vi "TazeASharg.vi"() -> ()   [LabVIEW 2022 SP3]
uses:
  StopControl.ctl
  StartControl.ctl
  ScoreIndicator.ctl
  TimeControl.ctl
  ComboIndicator.ctl
  NameControl.ctl
  FullHighscoreIndicator.ctl
  HighscoreIndicator.ctl
  FullHighScoreScoreIndicator.ctl
  HighscoreIndicatorYes.ctl
  ShargStates.ctl
  ShargTypeDef.ctl
  <vilib>/numeric/Random Number (Range) U64.vi
  <vilib>/numeric/sub_Random U32.vi
  <vilib>/MakerHub/LINX/Public/Utilities/Open Serial.vi
  <vilib>/MakerHub/LINX/Public/Sensors/Motion/Servo/Servo Open One Channel.vi
  <vilib>/MakerHub/LINX/Public/Sensors/Motion/Servo/Servo Close One Channel.vi
  <vilib>/MakerHub/LINX/LMH-LINX.lvlib
  <vilib>/MakerHub/LINX/Public/Sensors/Motion/Servo/Servo.lvlib
panel:
  out "High Score Scores":T1 caption="HIGH SCORE"
  out "High Score Names":T3 caption="HIGH SCORE"
  in  "Name":T5 caption="NAME"
  out "Overheat":bool
  out "COMBO":T6 format="%01d"
  out "TIME":T7 format="%02d"
  out "Hit?":bool
  out "SCORE":T8 format="%04d"
  in  "Start Game":T9
  in  "Stop Button":T10
  out "Energy":dbl(knob) caption="LASER ENERGY" scale=0.0..180.0
  # "HIGH SCORE"
  # "1."
  # "2."
  # "3."
  # "4."
  # "5."
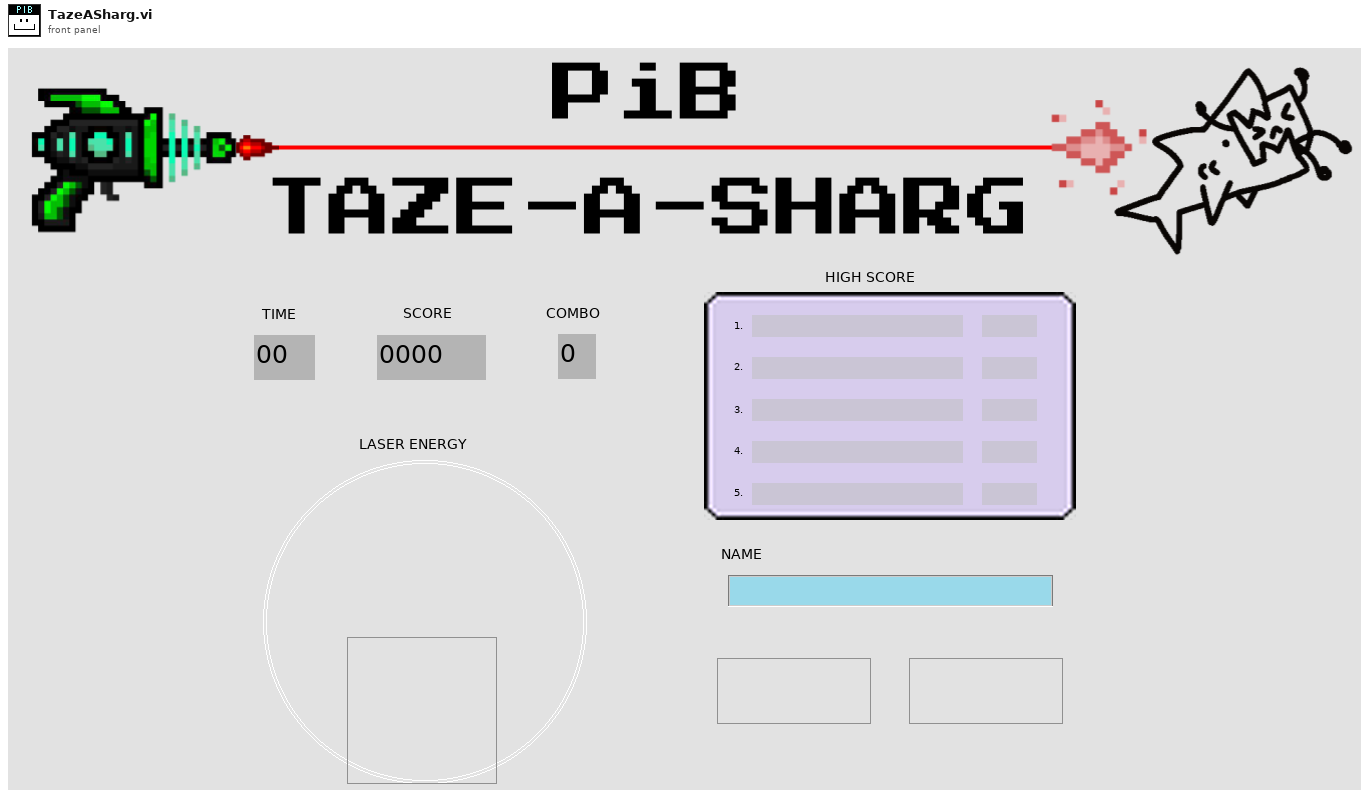
[diagram p1: front panel]
types:
  T1 = typedef "FullHighScoreScoreIndicator.ctl" = T2[]
  T2 = typedef "HighscoreIndicatorYes.ctl" = string
  T3 = typedef "FullHighscoreIndicator.ctl" = T4[]
  T4 = typedef "HighscoreIndicator.ctl" = string
  T5 = typedef "NameControl.ctl" = string
  T6 = typedef "ComboIndicator.ctl" = u32
  T7 = typedef "TimeControl.ctl" = u32
  T8 = typedef "ScoreIndicator.ctl" = u32
  T9 = typedef "StartControl.ctl" = bool
  T10 = typedef "StopControl.ctl" = bool
  T11 = cluster{"Target Up":bool, "Target Start Time":u32, "Target Up Time":u64, "Current Target":u64}
  T12 = cluster{"Laser Pin":u8, "Trigger Pin":u8, "Servo Pin":u8, "Photoresistor Pins":u8[], "RGB LED Pins":u8[]}
  T13 = typedef "ShargStates.ctl" = enum16{"Initialization", "Leaderboard", "Start Game", "Gameplay", "Update Final Score"}
  T14 = typedef "LMH-LINX.lvlib/LINX Ref.ctl" = cluster{"IO":T15, "Interface":T16, "LINX Device Config":T17}
  T15 = typedef "LMH-LINX.lvlib/Platform.ctl" = enum16{"Remote", "Local"}
  T16 = typedef "LMH-LINX.lvlib/Interface.ctl" = enum16{"Serial", "TCP"}
  T17 = typedef "LMH-LINX.lvlib/Device.lvlib/LINX Device Config.ctl" = cluster{"Interface":T16, "COM Port":refnum<visa-resource-name>, "TCP Configuration":T18, "Device Family":u8, "Device ID":u8, "Device Name":string, "TCP Ref":refnum<k5>, "Channels":T19}
  T18 = typedef "LMH-LINX.lvlib/Device.lvlib/TCP Config.ctl" = cluster{"IP Address":string, "Port":u16}
  T19 = typedef "LMH-LINX.lvlib/Channels.ctl" = cluster{"DI":u8[], "DO":u8[], "AI":u8[], "AO":u8[], "PWM":u8[], "QE":u8[], "UART":u8[], "I2C 2":u8[], "SPI":u8[], "CAN":u8[], "Servo":u8[], "AI Ref (V)":dbl, "AI Resolution (Bits)":u8, "AO Ref (V)":dbl, "AO Resolution (Bits)":u8}
  T20 = cluster{"Target Up":bool, "millisecond timer value":u32, "number":u64, "Current Target":u64}
  T21 = enum16{"open", "open or create", "create or replace", "create", "open (read-only)"}
  T22 = typedef "ShargTypeDef.ctl" = cluster{"Start Time":u32, "Score":u32, "Combo":u32, "RisingEdge":u32, "FallingEdge":u32, "Duration":u32, "Signal":i16, "NewTarget?":bool, "Username":string, "LastChannel":i32}
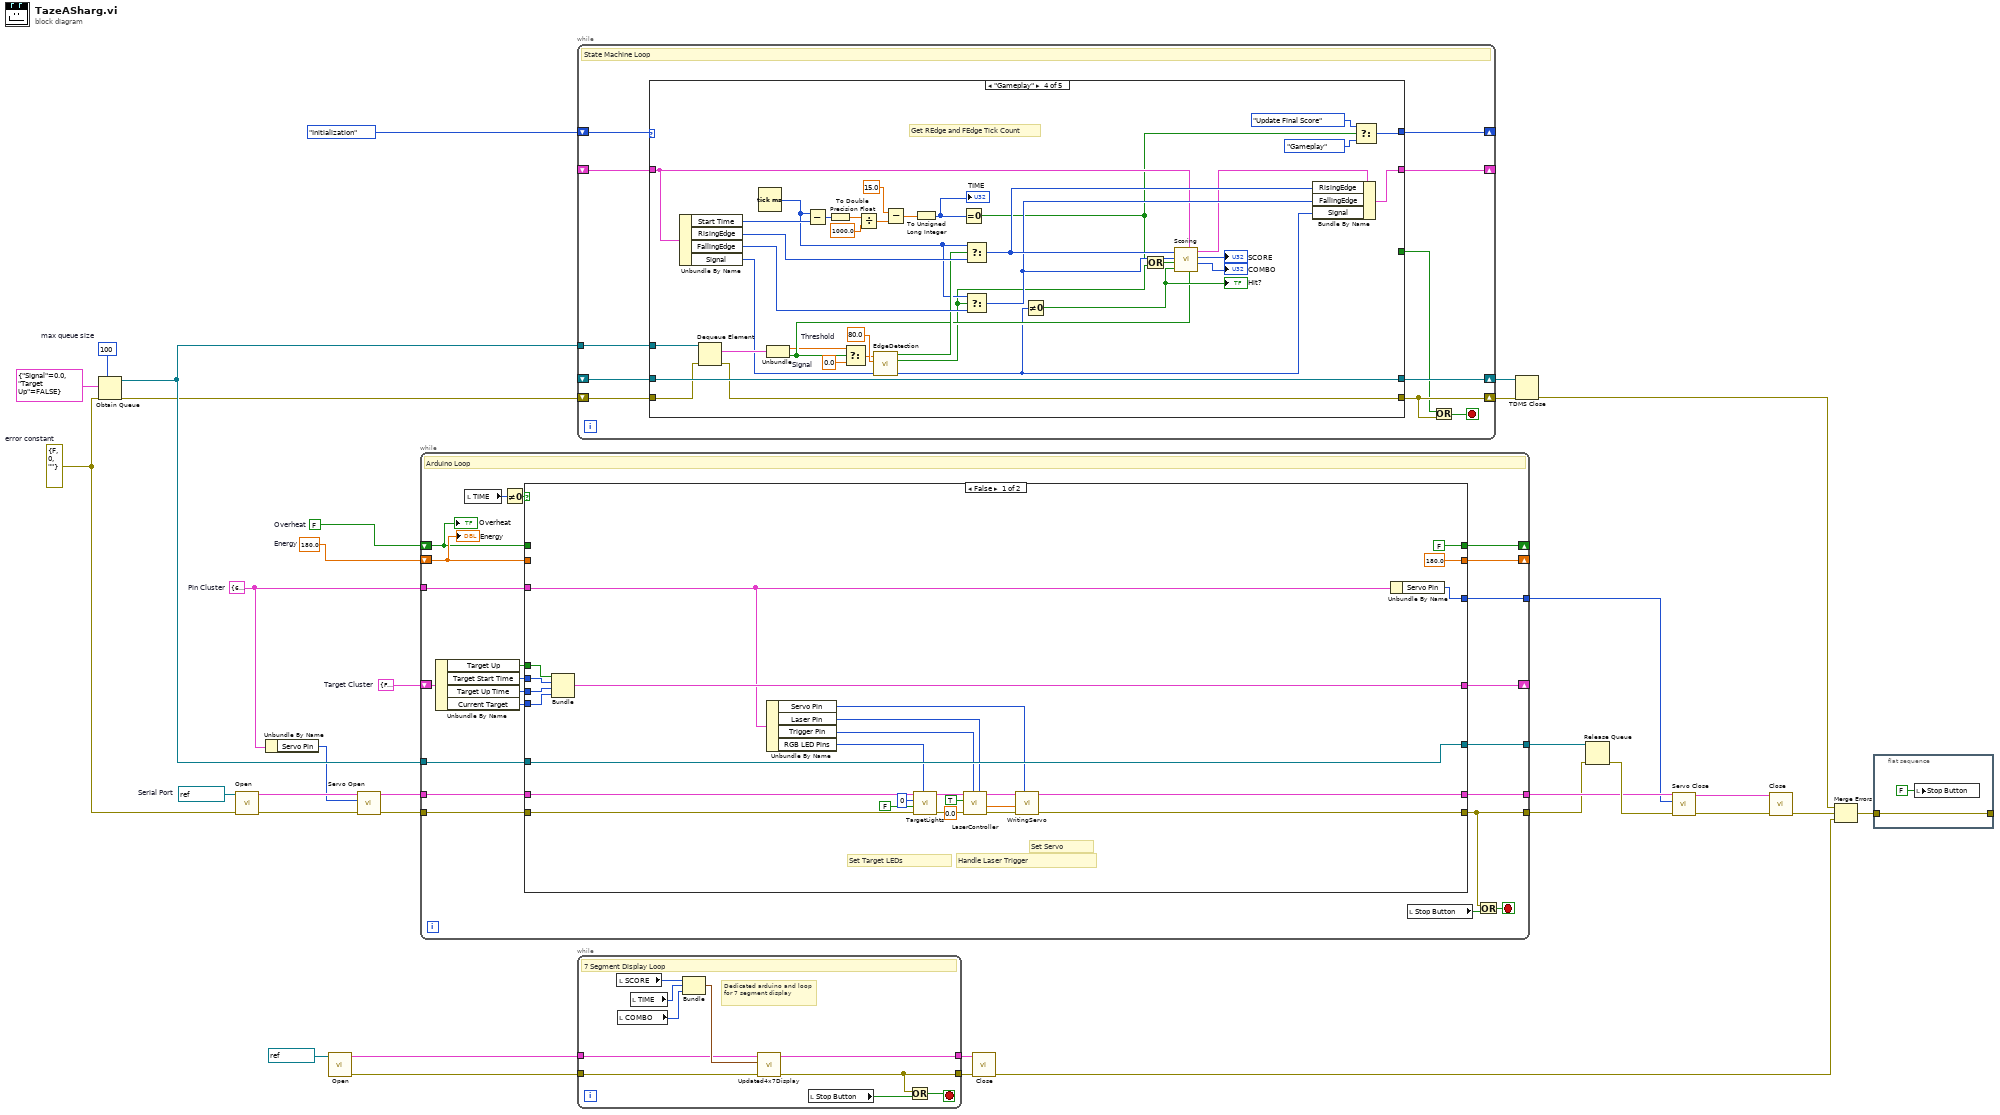
[diagram p0: block diagram]
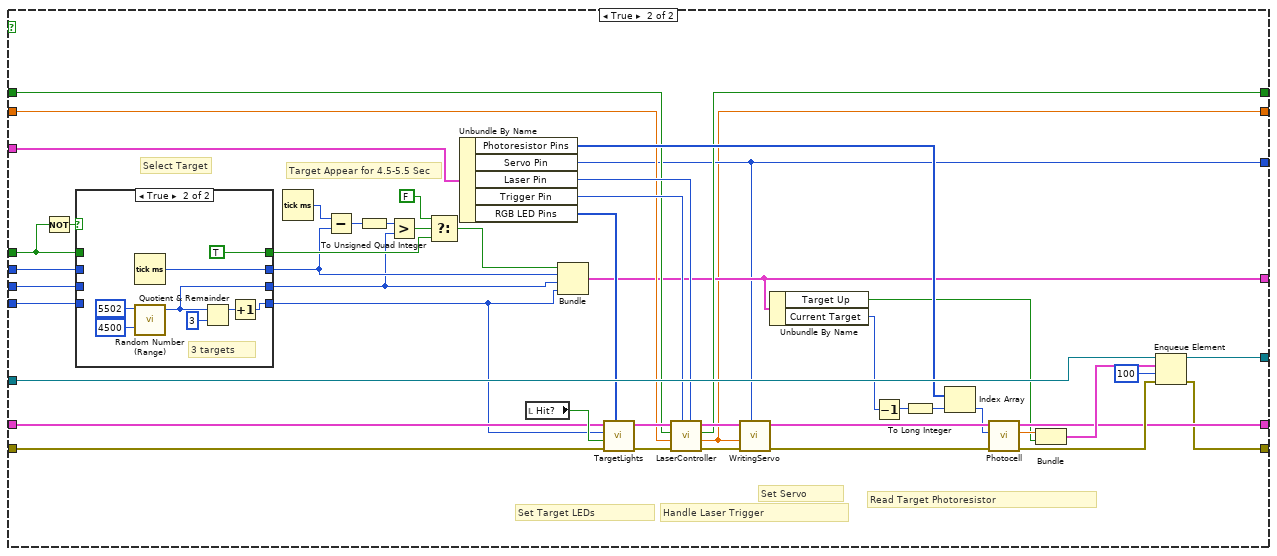
[diagram p2: hidden frame]
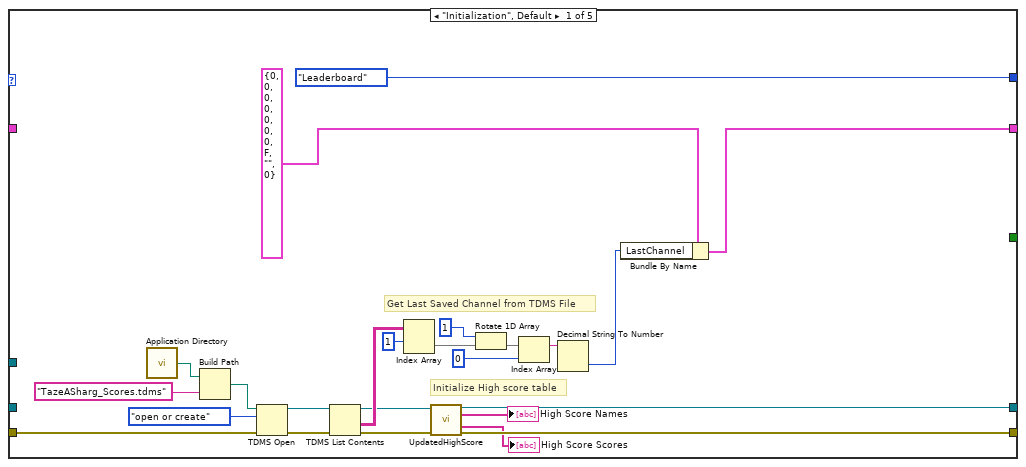
[diagram p4: hidden frame]
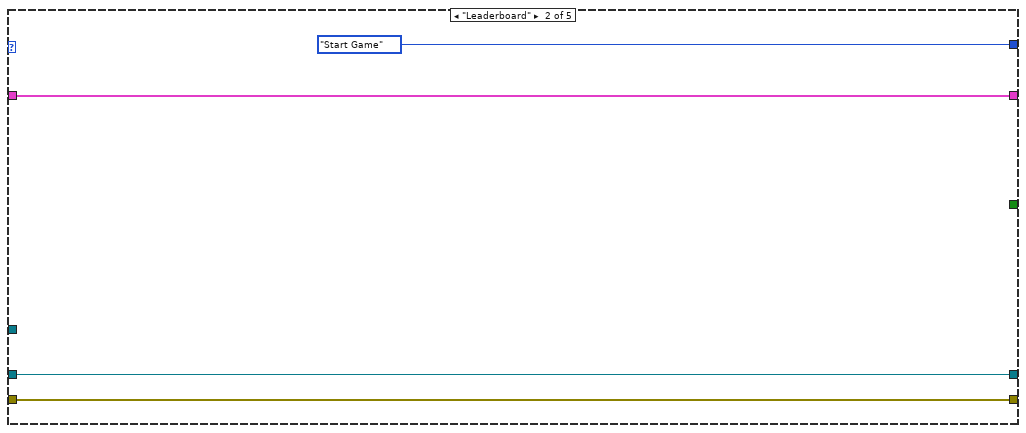
[diagram p5: hidden frame]
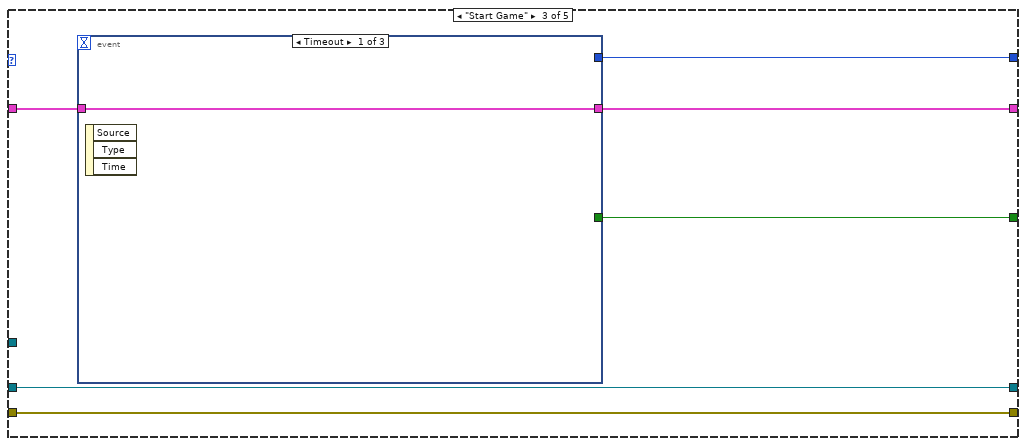
[diagram p6: hidden frame]
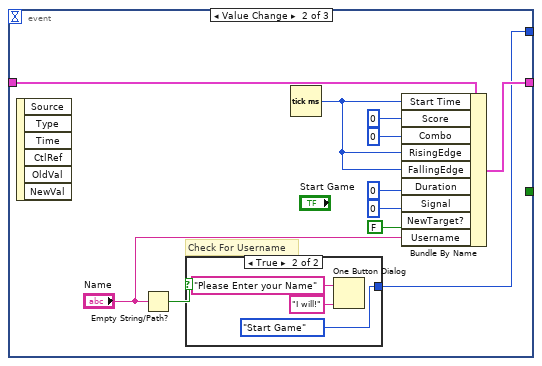
[diagram p7: hidden frame]
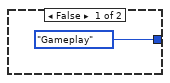
[diagram p8: hidden frame]
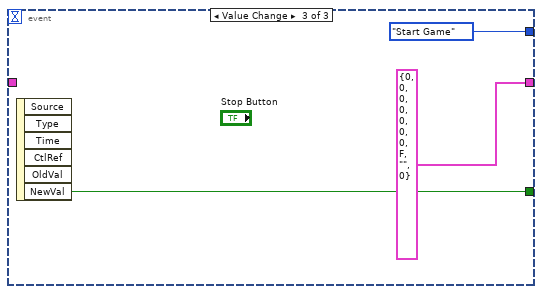
[diagram p9: hidden frame]
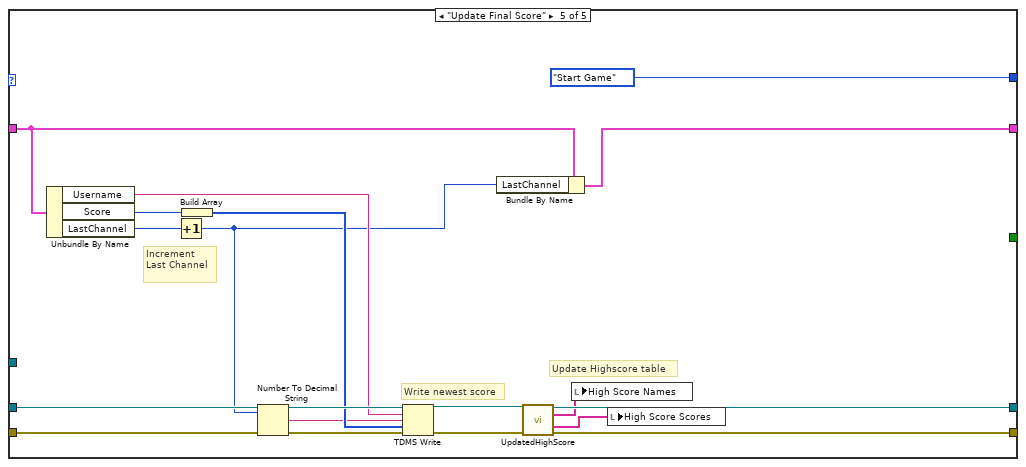
[diagram p10: hidden frame]
diagram:
  w5 = T11 {"Target Up"=FALSE, "Target Start Time"=0, "Target Up Time"=0, "Current Target"=0}  # Target Cluster
  w8 = 180.0  # Energy
  w9 = FALSE  # Overheat
  w2 = T12 {"Laser Pin"=6, "Trigger Pin"=3, "Servo Pin"=5, "Photoresistor Pins"=[0, 1, 2], "RGB LED Pins"=[22, 23, 24, 25, 26, 27]}  # Pin Cluster
  w30 = refnum<visa-resource-name> "COM8"  # Serial Port
  w31 = 100  # max queue size
  w10 = errorcluster {"status"=FALSE, "code"=0, "source"=""}  # error constant
  n1 = Obtain Queue(max queue size (-1, unlimited)=w31, element data type=cluster{"Signal":dbl, "Target Up":bool} {"Signal"=0.0, "Target Up"=FALSE}, error in (no error)=w10) -> (queue out=w33:refnum<queue>, error out=w11:errorcluster)  [unwired: 2 in, 1 out]
  n2 = call-poly <vilib>:"Open.vi"("Error In"=w10, "Serial Port"=w30) -> ("Error Out"=w27:errorcluster, "LINX Resource"=w29:T14)  [unwired: 7 in, 1 out]
  n3 = Unbundle By Name(w2) -> ("Servo Pin"=w1:u8)
  n4 = call-poly <vilib>:"Open.vi"("Serial Port"=refnum<visa-resource-name> "COM5") -> ("Error Out"=w20:errorcluster, "LINX Resource"=w21:T14)  [unwired: 8 in, 1 out]
  n5 = call-poly <vilib>:"Servo Open.vi"("Error In"=w27, "Servo Channel"=w1, "LINX Resource"=w29) -> ("Error Out"=w26:errorcluster, "LINX Resource"=w28:T14)  [unwired: 7 in]
  n6 = while {
    tunnel: w26 -> [w51]
    tunnel: w28 -> [w52]
    shift-right: [w48] -> _
    shift-left: w9 -> [w45]
    shift-right: [w47] -> _
    shift-left: w8 -> [w46]
    tunnel: w33 -> [w50]
    tunnel: w2 -> [w49]
    tunnel: [w44] -> w7
    tunnel: [w35] -> w3
    tunnel: [w43] -> w6
    shift-right: [w37] -> _
    shift-left: w5 -> [w42]
    tunnel: [w36] -> w4
    stop <- w54 stop-if-true
    # "Arduino Loop"
    n7 = Unbundle By Name(w42) -> ("Target Up"=w41:bool, "Target Start Time"=w40:u32, "Target Up Time"=w39:u64, "Current Target"=w38:u64)
    n8 = local read "TIME"() -> (w56:T7)
    n9 = Not Equal To 0?(x=w56) -> (x != 0?=w55:bool)
    n10 = case shown="False" w55 {
      tunnel: w40 -> [w79 w126]
      tunnel: w41 -> [w80 w125]
      tunnel: w38 -> [w77 w124]
      tunnel: w39 -> [w78 w123]
      tunnel: w52 -> [w66 w107]
      tunnel: w51 -> [w65 w106]
      tunnel: [w68 w105] -> w44
      tunnel: [w67 w104] -> w35
      tunnel: w50 -> [w81 w103]
      tunnel: w49 -> [w64 w101]
      tunnel: w46 -> [_ w96]
      tunnel: w45 -> [_ w95]
      tunnel: [FALSE ("Overheat Out") w94] -> w48
      tunnel: [180.0 ("Energy Out") w84] -> w47
      tunnel: [w81 w93] -> w43
      tunnel: [w76 w88] -> w37
      tunnel: [w75 w86] -> w36
      frame False {
        # "Set Servo"
        # "Handle Laser Trigger"
        # "Set Target LEDs"
        n11 = Bundle("Target Up"=w80, "Target Start Time"=w79, "Target Up Time"=w78, "Current Target"=w77) -> (w76:T11)  [unwired: 1 in]
        n12 = Unbundle By Name(w64) -> ("Servo Pin"=w60:u8, "Laser Pin"=w61:u8, "Trigger Pin"=w62:u8, "RGB LED Pins"=w63:u8[])
        n13 = call "TargetLights.vi"("DO Channels"=w63, "Error In"=w65, "Hit?"=FALSE, "Target Number"=u64 0, "LINX Resource"=w66) -> ("Error Out"=w71:errorcluster, "LINX Resource 2"=w72:T14)  [unwired: 5 in]
        n14 = call "LaserController.vi"("Laser Pin"=w61, "Trigger Pin"=w62, "Error In"=w71, "Energy In"=0.0, "Overheat In"=TRUE, "LINX Resource In"=w72) -> ("Error Out"=w74:errorcluster, "Energy Out"=w69:dbl, "LINX Resource Out"=w73:T14)  [unwired: 2 in, 1 out]
        n15 = call "WritingServo.vi"("Servo Pin"=w60, "error in (no error)"=w74, "Position"=w69, "LINX Resource in"=w73) -> ("error out"=w67:errorcluster, "LINX Resource out"=w68:T14)  [unwired: 6 in]
        n16 = Unbundle By Name(w64) -> ("Servo Pin"=w75:u8)
      }
      frame True {
        # "Set Servo"
        # "Read Target Photoresistor"
        # "Handle Laser Trigger"
        # "Set Target LEDs"
        # "Target Appear for 4.5-5.5 Sec"
        # "Select Target"
        n17 = Not(x=w125) -> (.not. x?=w122:bool)
        n18 = case shown="True" w122 {
          tunnel: [w134 TRUE] -> w128
          tunnel: [w135 w142] -> w91
          tunnel: [w133 w137] -> w89
          tunnel: w126 -> [w135 _]
          tunnel: w125 -> [w134 _]
          tunnel: w124 -> [w133 _]
          tunnel: [w132 w136] -> w90
          tunnel: w123 -> [w132 _]
          frame False {
          }
          frame True {
            # "3 targets"
            n19 = Tick Count (ms)() -> (millisecond timer value=w142:u32)
            n20 = call-poly <vilib>:"Random Number (Range).vi"("lower bound (0)"=u64 4500, "upper bound (100)"=u64 5502) -> ("number"=w136:u64)  [unwired: 9 in]
            n21 = Quotient & Remainder(x=w136, y=u64 3) -> (x-y*floor(x/y)=w139:u64)  [unwired: 1 out]
            n22 = Increment(x=w139) -> (x+1=w137:u64)
          }
        }
        n23 = Tick Count (ms)() -> (millisecond timer value=w131:u32)
        n24 = Subtract(x=w131, y=w91) -> (x-y=w130:u32)
        n25 = To Unsigned Quad Integer(1:w130) -> (0:w121:u64)
        n26 = Greater?(x=w121, y=w90) -> (0:w129:bool)
        n27 = Select(t=FALSE, s=w129, f=w128) -> (s? t:f=w92:bool)
        n28 = Unbundle By Name(w101) -> ("Photoresistor Pins"=w97:u8[], "Servo Pin"=w86:u8, "Laser Pin"=w98:u8, "Trigger Pin"=w99:u8, "RGB LED Pins"=w100:u8[])
        n29 = local read "Hit?"() -> (w114:bool)
        n30 = Bundle("Target Up"=w92, "millisecond timer value"=w91, "number"=w90, "Current Target"=w89) -> (w88:T20)  [unwired: 1 in]
        n31 = call "TargetLights.vi"("DO Channels"=w100, "Error In"=w106, "Hit?"=w114, "Target Number"=w89, "LINX Resource"=w107) -> ("Error Out"=w111:errorcluster, "LINX Resource 2"=w112:T14)  [unwired: 5 in]
        n32 = call "LaserController.vi"("Laser Pin"=w98, "Trigger Pin"=w99, "Error In"=w111, "Energy In"=w96, "Overheat In"=w95, "LINX Resource In"=w112) -> ("Error Out"=w120:errorcluster, "Energy Out"=w84:dbl, "Overheat Out"=w94:bool, "LINX Resource Out"=w119:T14)  [unwired: 2 in]
        n33 = call "WritingServo.vi"("Servo Pin"=w86, "error in (no error)"=w120, "Position"=w84, "LINX Resource in"=w119) -> ("error out"=w117:errorcluster, "LINX Resource out"=w116:T14)  [unwired: 6 in]
        n34 = Unbundle By Name(w88) -> ("Target Up"=w85:bool, "Current Target"=w87:u64)
        n35 = Decrement(x=w87) -> (x-1=w115:u64)
        n36 = To Long Integer(number=w115) -> (32bit integer=w113:i32)
        n37 = Index Array(array=w97, index=w113) -> (element=w102:u8)
        n38 = call <vilib>:"Photocell.vi"("Error In"=w117, "AI Channel"=w102, "LINX Resource"=w116) -> ("Error Out"=w118:errorcluster, "Value (0-100)"=w109:dbl, "LINX Resource"=w105:T14)  [unwired: 6 in]
        n39 = Bundle("Value (0-100)"=w109, "Target Up"=w85) -> (w110:cluster{"Value (0-100)":dbl, "Target Up":bool})  [unwired: 1 in]
        n40 = Enqueue Element(queue=w103, element=w110, timeout in ms (-1)=100, error in (no error)=w118) -> (queue out=w93:refnum<queue>, error out=w104:errorcluster)  [unwired: 1 out]
      }
    }
    n41 = local read "Stop Button"() -> (w53:T10)
    n42 = Or(x=w35, y=w53) -> (x .or. y?=w54:T10)
    "Overheat" <- w45
    "Energy" <- w46
  }
  n43 = while {
    shift-right: [w153] -> _
    shift-left: ShargStates."Initialization" -> [w154]
    shift-right: [w152] -> _
    shift-left: _ -> [w151]
    tunnel: w33 -> [w150]
    shift-right: [w148] -> w17
    shift-left: _ -> [w147]
    shift-right: [w145] -> w16
    shift-left: w11 -> [w146]
    stop <- w149 stop-if-true
    # "State Machine Loop"
    n44 = case shown="\"Gameplay\"" w154 {
      tunnel: [ShargStates."Leaderboard" ShargStates."Start Game" w188 w245 ShargStates."Start Game"] -> w153
      tunnel: [w157 w181 w186 w208 w246] -> w152
      tunnel: w151 -> [_ w181 w187 w233 w248]
      tunnel: w150 -> [_ _ _ w242 _]
      tunnel: [w160 w179 w185 w209 w252] -> w145
      tunnel: [w161 w180 w183 w214 w253] -> w148
      tunnel: w147 -> [_ w180 w183 w214 w261]
      tunnel: w146 -> [w174 w179 w185 w210 w260]
      tunnel: [_ _ w184 _ _] -> w144
      frame "Initialization", Default {
        # "Get Last Saved Channel from TDMS File"
        # "Initialize High score table"
        n45 = call <vilib>:"Application Directory.vi"() -> ("Application Directory"=w177:path)
        n46 = Build Path(base path=w177, name or relative path="TazeASharg_Scores.tdms") -> (appended path=w176:path)
        n47 = TDMS Open(8:w174, 10:T21."open or create" ("operation (0:open)"), 11:w176) -> (0:w172:errorcluster, 3:w173:refnum<k34>)  [unwired: 4 in]
        n48 = TDMS List Contents(4:w172, 7:w173) -> (0:w159:errorcluster, 1:w166:string[][], 3:w162:refnum<k34>)  [unwired: 1 in, 1 out]
        n49 = Index Array(array=w166, index (row)=1) -> (element=w171:string[])  [unwired: 1 in]
        n50 = call "UpdatedHighScore.vi"("tdms file"=w162, "error in (no error)"=w159) -> ("tdms file out"=w161:refnum<k34>, "Names"=→"High Score Names":string[], "Scores"=→"High Score Scores":string[], "error out"=w160:errorcluster)  [unwired: 10 in]
        n51 = Rotate 1D Array(1:w171, 2:1 ("n")) -> (0:w169:string[])
        n52 = Index Array(array=w169, index=0) -> (element=w165:string)
        n53 = Decimal String To Number(string=w165) -> (number=w163:i32)  [unwired: 2 in, 1 out]
        n54 = Bundle By Name(cluster=T22 {"Start Time"=0, "Score"=0, "Combo"=0, "RisingEdge"=0, "FallingEdge"=0, "Duration"=0, "Signal"=0, "NewTarget?"=FALSE, "Username"="", "LastChannel"=0} ("Cluster"), "LastChannel"=w163) -> (w157:T22)
      }
      frame "Leaderboard" {
      }
      frame "Start Game" {
        n55 = event shown="[0] Timeout" {
          selector: _ -> [_ _ _]
          dyn-events: _ -> [_ _ _]
          timeout: _ -> [_ _ _]
          tunnel: [_ w191 ShargStates."Start Game"] -> w188
          tunnel: w187 -> [w189 w200 _]
          tunnel: [w189 w199 T22 {"Start Time"=0, "Score"=0, "Combo"=0, "RisingEdge"=0, "FallingEdge"=0, "Duration"=0, "Signal"=0, "NewTarget?"=FALSE, "Username"="", "LastChannel"=0} ("Cluster Out")] -> w186
          tunnel: [_ _ w205] -> w184
          event Timeout {
            n56 = event-data() -> ()  [unwired: 1 in, 3 out]
          }
          event Value Change {
            # "Check For Username"
            n57 = event-data() -> ()  [unwired: 1 in, 6 out]
            n58 = Empty String/Path?(string/path="Name") -> (empty?=w192:bool)
            n59 = case shown="True" w192 {
              tunnel: [ShargStates."Gameplay" ShargStates."Start Game"] -> w191
              frame False {
              }
              frame True {
                n60 = One Button Dialog(message="Please Enter your Name", button name ("OK")="I will!") -> ()  [unwired: 1 out]
              }
            }
            n61 = Tick Count (ms)() -> (millisecond timer value=w193:u32)
            n62 = Bundle By Name(cluster=w200, "Start Time"=w193, "Score"=u32 0, "Combo"=u32 0, "RisingEdge"=w193, "FallingEdge"=w193, "Duration"=u32 0, "Signal"=i16 0, "NewTarget?"=FALSE, "Username"="Name") -> (w199:T22)
          }
          event Value Change {
            n63 = event-data() -> ("NewVal"=w205:T10)  [unwired: 1 in, 5 out]
          }
        }
      }
      frame "Gameplay" {
        w235 = 0.0  # Signal
        w241 = 80.0  # Threshold
        # "Get REdge and FEdge Tick Count"
        n64 = Unbundle By Name(w233) -> ("Start Time"=w231:u32, "RisingEdge"=w238:u32, "FallingEdge"=w237:u32, "Signal"=w217:i16)
        n65 = Dequeue Element(queue=w242, error in (no error)=w210) -> (element=w232:cluster{"Signal":dbl, "Target Up":bool}, error out=w209:errorcluster)  [unwired: 1 in, 2 out]
        n66 = Tick Count (ms)() -> (millisecond timer value=w230:u32)
        n67 = Unbundle(w232) -> ("Signal"=w219:dbl, "Target Up"=w220:bool)
        n68 = Subtract(x=w230, y=w231) -> (x-y=w229:u32)
        n69 = To Double Precision Float(number=w229) -> (double precision float=w227:dbl)
        n70 = Select(t=w219, s=w220, f=w235) -> (s? t:f=w218:dbl)
        n71 = Divide(x=w227, y=1000.0) -> (x/y=w226:dbl)
        n72 = call "EdgeDetection.vi"("Previous Value"=w217, "Threshold"=w241, "Analog Input"=w218) -> ("Digitized"=w216:i16, "Falling Edge"=w212:bool, "Rising Edge"=w236:bool)  [unwired: 4 in]
        n73 = Subtract(x=15.0, y=w226) -> (x-y=w222:dbl)
        n74 = To Unsigned Long Integer(number=w222) -> (unsigned 32bit integer=w215:u32)
        "TIME" <- w215
        n75 = Equal To 0?(x=w215) -> (x = 0?=w213:bool)
        n76 = Select(t=w230, s=w236, f=w238) -> (s? t:f=w240:u32)
        n77 = Select(t=w230, s=w212, f=w237) -> (s? t:f=w239:u32)
        n78 = Not Equal To 0?(x=w216) -> (x != 0?=w221:bool)
        "Hit?" <- w221
        n79 = Or(x=w213, y=w212) -> (x .or. y?=w211:bool)
        n80 = call "Scoring.vi"("RisingEdge"=w240, "FallingEdge"=w239, "FallingEdge?"=w211, "Hit?"=w221, "Cluster In"=w233, "TargetUp?"=w220) -> ("Cluster Out"=w234:T22, "Live Score"=→"SCORE":u32, "Combo"=→"COMBO":u32)  [unwired: 2 in]
        n81 = Bundle By Name(cluster=w234, "RisingEdge"=w240, "FallingEdge"=w239, "Signal"=w216) -> (w208:T22)
        n82 = Select(t=ShargStates."Update Final Score", s=w213, f=ShargStates."Gameplay") -> (s? t:f=w245:T13)
      }
      frame "Update Final Score" {
        # "Write newest score"
        # "Update Highscore table"
        # "Increment Last Channel"
        n83 = Unbundle By Name(w248) -> ("Username"=w256:string, "Score"=w259:u32, "LastChannel"=w255:i32)
        n84 = Increment(x=w255) -> (x+1=w247:i32)
        n85 = Build Array(w259) -> (w258:u32[])
        n86 = Number To Decimal String(number=w247) -> (decimal integer string=w257:string)  [unwired: 1 in]
        n87 = TDMS Write(0:w261, 5:w256, 7:w257, 9:w258, 11:w260) -> (4:w254:refnum<k34>, 15:w251:errorcluster)  [unwired: 1 in, 2 out]
        n88 = Bundle By Name(cluster=w248, "LastChannel"=w247) -> (w246:T22)
        n89 = call "UpdatedHighScore.vi"("tdms file"=w254, "error in (no error)"=w251) -> ("tdms file out"=w253:refnum<k34>, "Names"=w250:string[], "Scores"=w249:string[], "error out"=w252:errorcluster)  [unwired: 10 in]
        n90 = local write "High Score Names"(w250) -> ()
        n91 = local write "High Score Scores"(w249) -> ()
      }
    }
    n92 = Or(x=w144, y=w145) -> (x .or. y?=w149:T10)
  }
  n93 = while {
    tunnel: w21 -> [w268]
    tunnel: w20 -> [w267]
    tunnel: [w266] -> w19
    tunnel: [w264] -> w18
    stop <- w265 stop-if-true
    # "Dedicated arduino and loop for 7 segment display"
    # "7 Segment Display Loop"
    n94 = local read "SCORE"() -> (w272:T8)
    n95 = local read "COMBO"() -> (w270:T6)
    n96 = local read "TIME"() -> (w271:T7)
    n97 = Bundle("SCORE"=w272, "TIME"=w271, "COMBO"=w270) -> (w269:cluster{"SCORE":T8, "TIME":T7, "COMBO":T6})  [unwired: 1 in]
    n98 = call "Updated4x7Display.vi"("Error In"=w267, "Cluster"=w269, "LINX Resource In"=w268) -> ("Error Out"=w264:errorcluster, "LINX Resource Out"=w266:T14)  [unwired: 7 in]
    n99 = local read "Stop Button"() -> (w263:T10)
    n100 = Or(x=w264, y=w263) -> (x .or. y?=w265:T10)
  }
  n101 = call <vilib>:"Close.vi"("Error In"=w18, "LINX Resource"=w19) -> ("Error Out"=w12:errorcluster)  [unwired: 9 in]
  n102 = TDMS Close(8:w16, 11:w17) -> (0:w13:errorcluster)  [unwired: 1 out]
  n103 = Release Queue(queue=w6, error in (no error)=w3) -> (error out=w23:errorcluster)  [unwired: 1 in, 2 out]
  n104 = call-poly <vilib>:"Servo Close.vi"("Error In"=w23, "Servo Channel"=w4, "LINX Resource"=w7) -> ("Error Out"=w24:errorcluster, "LINX Resource"=w25:T14)  [unwired: 7 in]
  n105 = call <vilib>:"Close.vi"("Error In"=w24, "LINX Resource"=w25) -> ("Error Out"=w15:errorcluster)  [unwired: 9 in]
  n106 = Merge Errors(w13, w15, w12) -> (w14:errorcluster)
  n107 = flat-sequence {
    tunnel: w14 -> [w273]
    tunnel: [w273] -> _
    frame #0 {
      n108 = local write "Stop Button"(FALSE ("Stop Button")) -> ()
    }
  }
